vi "ReadData.vi"(8 "error in":errorcluster, 11 "Module Config Selector":i16) -> (0 "error out":errorcluster, 3 "Data Array":sgl[](array[numeric]) format="%.2f")   [LabVIEW 2017, in "BOP_VibAPI_2.lvlib"]
uses:
  <vilib>/addons/InsightCM/Devices/Shared/Cms/Fpga/Acquisition/source/subVIs/VibAPI_2/BOP_VibAPI_2.lvlib
  <vilib>/rvi/eio/common/nirviEmuTemplateMethod_errors.vi
  <vilib>/eio/EIONode/EIONode.xnode
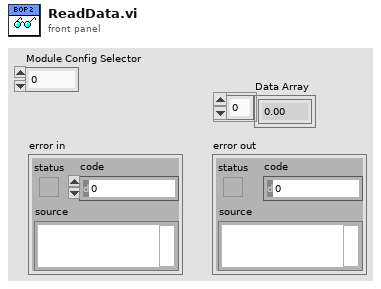
[diagram p1: front panel]
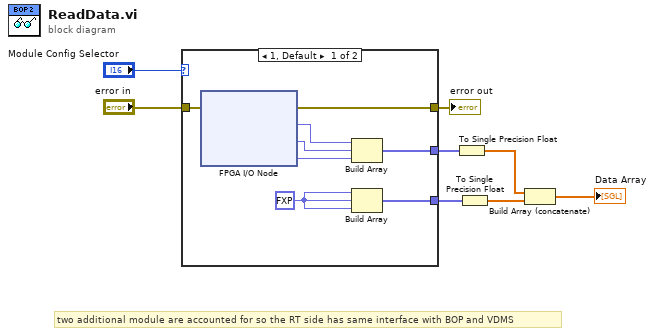
[diagram p0: block diagram]
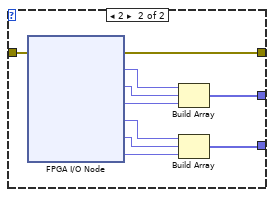
[diagram p2: hidden frame]
diagram:
  # "two additional module are accounted for so the RT side has same interface with BOP and VDMS"
  n1 = case shown="1, Default" "Module Config Selector" {
    tunnel: "error in" -> [w13 w23]
    tunnel: [w12 w22] -> w7
    tunnel: [w9 w18] -> w4
    tunnel: [w11 w17] -> w2
    frame 1, Default {
      w10 = fxp<+/-,24,7> 0.0 ("Mod1/AI2")
      n2 = xnode "FPGA I/O Node"("error in"=w13) -> ("error out"=w12:errorcluster, "Mod1/AI0"=w14:fxp<+/-,24,7>, "Mod1/AI1"=w16:fxp<+/-,24,7>, "Mod1/AI2"=w15:fxp<+/-,24,7>)  [unwired: 3 in, 3 out]
      n3 = Build Array(w14, w16, w15) -> (w9:fxp<+/-,24,7>[])
      n4 = Build Array(w10, w10, w10) -> (w11:fxp<+/-,24,7>[])
    }
    frame 2 {
      n5 = xnode "FPGA I/O Node"("error in"=w23) -> ("error out"=w22:errorcluster, "Mod1/AI0"=w24:fxp<+/-,24,7>, "Mod1/AI1"=w26:fxp<+/-,24,7>, "Mod1/AI2"=w25:fxp<+/-,24,7>, "Mod2/AI0"=w21:fxp<+/-,24,7>, "Mod2/AI1"=w20:fxp<+/-,24,7>, "Mod2/AI2"=w19:fxp<+/-,24,7>)  [unwired: 6 in, 6 out]
      n6 = Build Array(w24, w26, w25) -> (w18:fxp<+/-,24,7>[])
      n7 = Build Array(w21, w20, w19) -> (w17:fxp<+/-,24,7>[])
    }
  }
  "error out" <- w7
  n8 = To Single Precision Float(number=w4) -> (single precision float=w3:sgl[])
  n9 = To Single Precision Float(number=w2) -> (single precision float=w1:sgl[])
  n10 = Build Array (concatenate)(w3, w1) -> (→"Data Array":sgl[])
